vi "read1Byte Tx Rx.vi"(7 "address":u16, 9 "id":u8, 10 "protocol_version":i32, 11 "port_num":i32) -> (3 "function return":u8)   [LabVIEW 2016, in "dxl_x86_c.lvlib"]
doc: "WINDECLSPEC uint8_t read1ByteTxRx (int port_num, int protocol_version, uint8_t id, uint16_t address);"
uses:
  dxl_x86_c.lvlib
  dxl_x86_c.dll
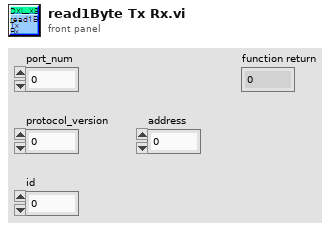
[diagram p1: front panel]
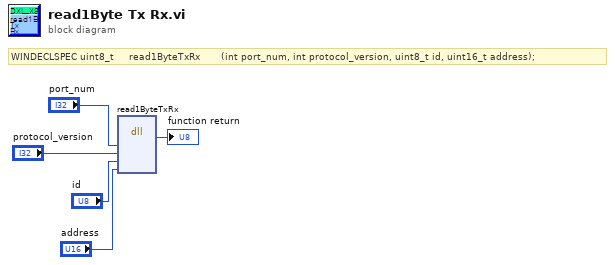
[diagram p0: block diagram]
diagram:
  # "WINDECLSPEC uint8_t     read1ByteTxRx       (int port_num, int protocol_version, uint8_t id, uint16_t address);"
  n1 = dll-call lib="C:/Users/Platform/Desktop/DynamixelSDK/labview/dxl_x86_c.lvlib/dxl_x86_c.*" fn="read1ByteTxRx"("port_num"="port_num", "protocol_version"="protocol_version", "id"="id", "address"="address") -> (→"function return":u8)  [unwired: 7 in, 2 out]
